vi "LiveCapture.vi"(8 "ErrorIn":errorcluster, 11 "OpenCVCamIn":refnum<class "OpenCVCam.lvclass">) -> (0 "ErrorOut":errorcluster, 3 "OpenCVCamOut":refnum<class "OpenCVCam.lvclass">)   [LabVIEW 2021, in "OpenCVCam.lvclass"]
uses:
  OpenCVCam.lvclass
  C:/Localdata/Projects/TriekselSoft/TriekselsoftApplicationFramework/Source/.Externals/Library_YAF/YActor/YActor.lvclass
  Library_YAF/YActor/ExeCmd_async.vi
  Library_YAF/YActor/YActor.lvclass
  C:/Localdata/Projects/TriekselSoft/TriekselsoftApplicationFramework/Source/.Externals/Library_YAF/YAFTAF/YAFTAF.lvclass
  C:/Localdata/Projects/TriekselSoft/TriekselsoftApplicationFramework/Source/.Externals/Interface_UserInterface_IFrontPanel/IFrontPanel/IFrontPanel.lvclass
  C:/Localdata/Projects/TriekselSoft/TriekselsoftApplicationFramework/Source/.Externals/Interface_TAF_IInterface/IInterface/IInterface.lvclass
  C:/Localdata/Projects/TriekselSoft/TriekselsoftApplicationFramework/Source/.Externals/Interface_Object_ICreateDestroy/ICreateDestroy/ICreateDestroy.lvclass
  C:/Localdata/Projects/TriekselSoft/TriekselsoftApplicationFramework/Source/.Externals/Interface_Object_IPersistentData/IPersistentData/IPersistentData.lvclass
  C:/Localdata/Projects/TriekselSoft/TriekselsoftApplicationFramework/Source/.Externals/Interface_TAF_ITAFObject/ITAFObject/ITAFObject.lvclass
  C:/Localdata/Projects/TriekselSoft/TriekselsoftApplicationFramework/Source/YAFTAFObjects/OpenCVCam/OpenCVCam.lvclass
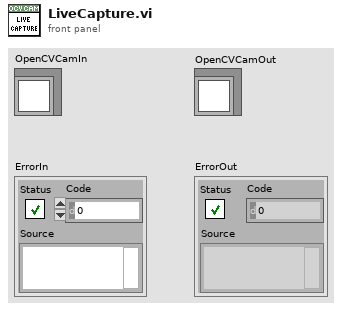
[diagram p1: front panel]
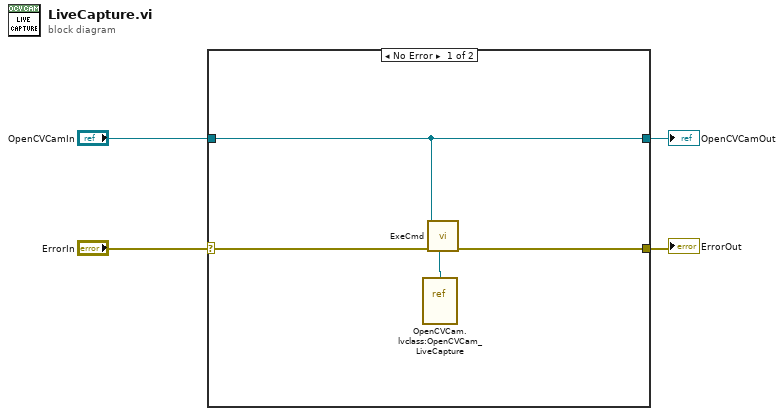
[diagram p0: block diagram]
diagram:
  n1 = case shown="No Error" "ErrorIn" {
    selector: "ErrorIn" -> [w8 w10]
    tunnel: [w7 w10] -> w3
    tunnel: [w5 w9] -> w1
    tunnel: "OpenCVCamIn" -> [w5 w9]
    frame No Error {
      n2 = vi-ref "OpenCVCam.lvclass:OpenCVCam_LiveCapture.vi"() -> (w6:refnum<vi>)
      n3 = call-poly "ExeCmd.vi"("CmdVIRef"=w6, "ErrorIn"=w8, "YActorIn"=w5) -> ("ErrorOut"=w7:errorcluster)  [unwired: 8 in]
    }
    frame Error {
    }
  }
  "ErrorOut" <- w3
  "OpenCVCamOut" <- w1
